vi "refresh group tree.vi"(8 "error in":errorcluster, 9 "channels":refnum<class "TBM channel.lvclass">[](array[class]), 10 "avail logged tags table":refnum<vi>, 11 "groups list":refnum<vi>) -> (0 "error out":errorcluster)   [LabVIEW 2015, in "TDMS datalogger editor node.lvclass"]
uses:
  TDMS datalogger editor node.lvclass
  <vilib>/NI/Tag Bus Module Framework/channel/TBM channel.lvclass
  <vilib>/NI/Tag Bus/tag/tag descriptor.lvclass/tag descriptor.ctl
  <vilib>/NI/Tag Bus/tag/tag descriptor.lvclass
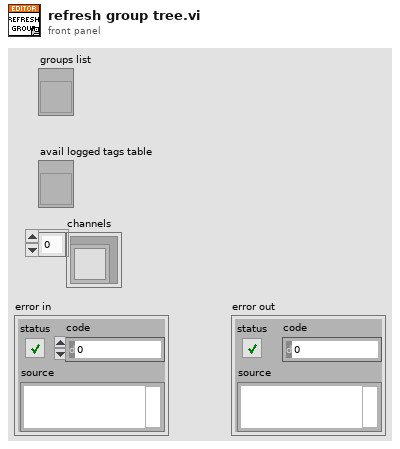
[diagram p1: front panel]
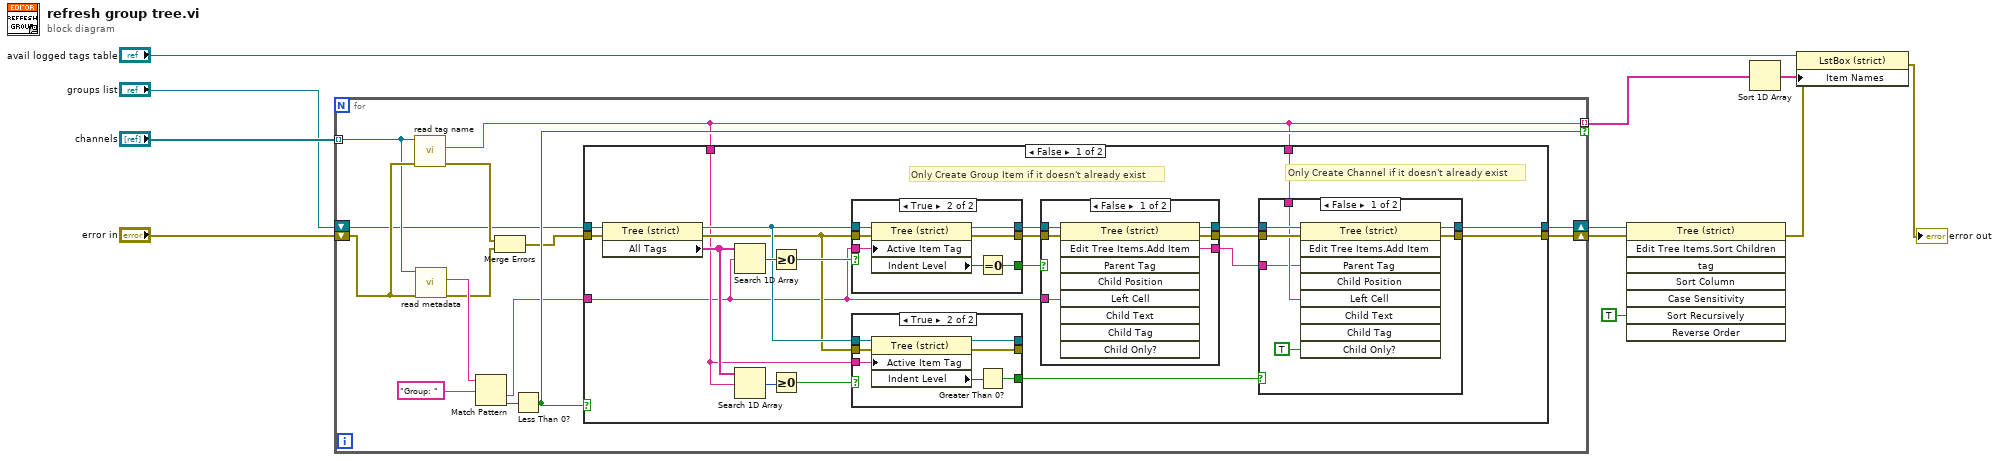
[diagram p0: block diagram]
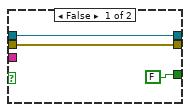
[diagram p3: hidden frame]
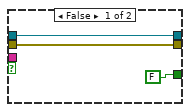
[diagram p5: hidden frame]
diagram:
  n1 = for {
    tunnel: [w12] -> w11 mode=indexing if=w23
    shift-right: [w22] -> w8
    shift-left: "error in" -> [w20]
    tunnel: "channels" -> [w15] mode=indexing
    shift-right: [w16] -> w6
    shift-left: "groups list" -> [w14]
    n2 = call <vilib>:"read tag name.vi"("error in"=w20, "system tag in"=w15) -> ("error out"=w19:errorcluster, "name"=w12:string)  [unwired: 7 in, 1 out]
    n3 = call <vilib>:"read metadata.vi"("error in"=w20, "system tag in"=w15) -> ("error out"=w17:errorcluster, "metadata"=w21:string)  [unwired: 7 in, 1 out]
    n4 = Match Pattern(string=w21, regular expression="Group: ") -> (after substring=w13:string, offset past match=w24:i32)  [unwired: 1 in, 2 out]
    n5 = Merge Errors(w19, w17) -> (w18:errorcluster)
    n6 = Less Than 0?(x=w24) -> (x < 0?=w23:bool)
    n7 = case shown="False" w23 {
      tunnel: w14 -> [w43 w85]
      tunnel: w13 -> [w26 _]
      tunnel: w12 -> [w44 _]
      tunnel: w18 -> [w37 w86]
      tunnel: [w35 w86] -> w22
      tunnel: [w34 w85] -> w16
      tunnel: w12 -> [w28 _]
      frame False {
        # "Only Create Channel if it doesn't already exist"
        # "Only Create Group Item if it doesn't already exist"
        n8 = property class="Tree (strict)"(reference=w43, error in=w37) -> (reference out=w30:refnum<vi>, error out=w29:errorcluster, "All Tags"=w33:string[])
        n9 = Search 1D Array(1D array=w33, element=w26) -> (index of element=w42:i32)  [unwired: 1 in]
        n10 = Search 1D Array(1D array=w33, element=w28) -> (index of element=w32:i32)  [unwired: 1 in]
        n11 = Greater Or Equal To 0?(x=w42) -> (x >= 0?=w41:bool)
        n12 = Greater Or Equal To 0?(x=w32) -> (x >= 0?=w31:bool)
        n13 = case shown="True" w41 {
          tunnel: w26 -> [_ w84]
          tunnel: [FALSE w82] -> w40
          tunnel: w30 -> [w77 w81]
          tunnel: [w77 w80] -> w39
          tunnel: [w75 w79] -> w38
          tunnel: w29 -> [w75 w78]
          frame False {
          }
          frame True {
            n14 = property class="Tree (strict)"(reference=w81, error in=w78, "Active Item Tag"=w84) -> (reference out=w80:refnum<vi>, error out=w79:errorcluster, "Indent Level"=w83:i32)
            n15 = Equal To 0?(x=w83) -> (x = 0?=w82:bool)
          }
        }
        n16 = case shown="True" w31 {
          tunnel: w28 -> [_ w65]
          tunnel: [FALSE w63] -> w27
          tunnel: w30 -> [w58 w62]
          tunnel: [w58 w61] -> _
          tunnel: [w56 w60] -> _
          tunnel: w29 -> [w56 w59]
          frame False {
          }
          frame True {
            n17 = property class="Tree (strict)"(reference=w62, error in=w59, "Active Item Tag"=w65) -> (reference out=w61:refnum<vi>, error out=w60:errorcluster, "Indent Level"=w64:i32)
            n18 = Greater Than 0?(x=w64) -> (x > 0?=w63:bool)
          }
        }
        n19 = case shown="False" w40 {
          tunnel: [w71 w73] -> w46
          tunnel: [w70 w72] -> w45
          tunnel: [w69 w74] -> w36
          tunnel: w26 -> [w68 w74]
          tunnel: w39 -> [w67 w72]
          tunnel: w38 -> [w66 w73]
          frame False {
            n20 = invoke class="Tree (strict)" method="Edit Tree Items.Add Item"(reference=w67, error in=w66, "Left Cell"=w68) -> (reference out=w70:refnum<vi>, error out=w71:errorcluster, "Edit Tree Items:Add Item"=w69:string)  [unwired: 6 in, 6 out]
          }
          frame True {
          }
        }
        n21 = case shown="False" w27 {
          tunnel: w46 -> [w53 w55]
          tunnel: w45 -> [w52 w54]
          tunnel: w44 -> [w51 _]
          tunnel: w36 -> [w49 _]
          tunnel: [w48 w55] -> w35
          tunnel: [w47 w54] -> w34
          frame False {
            n22 = invoke class="Tree (strict)" method="Edit Tree Items.Add Item"(reference=w52, error in=w53, "Parent Tag"=w49, "Left Cell"=w51, "Child Only?"=TRUE) -> (reference out=w47:refnum<vi>, error out=w48:errorcluster)  [unwired: 4 in, 7 out]
          }
          frame True {
          }
        }
      }
      frame True {
      }
    }
  }
  n23 = invoke class="Tree (strict)" method="Edit Tree Items.Sort Children"(reference=w6, error in=w8, "Sort Recursively"=TRUE ("Sort Recursively?")) -> (error out=w7:errorcluster)  [unwired: 5 in, 7 out]
  n24 = Sort 1D Array(array=w11) -> (sorted array=w1:string[])
  n25 = property on="Property Node" class="LstBox (strict)"(reference="avail logged tags table", error in=w7, "Item Names"=w1) -> (error out=→"error out":errorcluster)  [unwired: 1 out]
